vi "PMT imaging_ v1.vi"() -> ()   [LabVIEW 2012]
uses:
  <vilib>/DAQmx/write.llb/DAQmx Write (Analog 1D Wfm NChan NSamp).vi
  <vilib>/DAQmx/read.llb/DAQmx Read (Counter 1D U32 1Chan NSamp).vi
  <vilib>/DAQmx/create/channels.llb/DAQmx Create Channel (AO-Voltage-Basic).vi
  <vilib>/DAQmx/configure/timing.llb/DAQmx Timing (Sample Clock).vi
  <vilib>/DAQmx/configure/trigger.llb/DAQmx Start Trigger (Digital Edge).vi
  <vilib>/DAQmx/create/channels.llb/DAQmx Create Channel (CI-Count Edges).vi
  <vilib>/DAQmx/miscellaneous.llb/DAQmx Fill In Error Info.vi
  <resource>/objmgr/daqmx.rc
panel:
  in  "shift":i8
  in  "Normalization":dbl=255.0
  out "Output":dbl[](array[numeric])
  out "size(s)":i32
  out "data":u32[](array[numeric])
  out "Image":T1(plugin-control)
  out "Waveform Chart":dbl[](graph)
  in  "Exp Time (s)":dbl=4.0
  in  "Y line":i32=512
  in  "Y step (um)":dbl=0.1
  in  "X step (um)":dbl=0.1
  in  "X pixel":i32=512
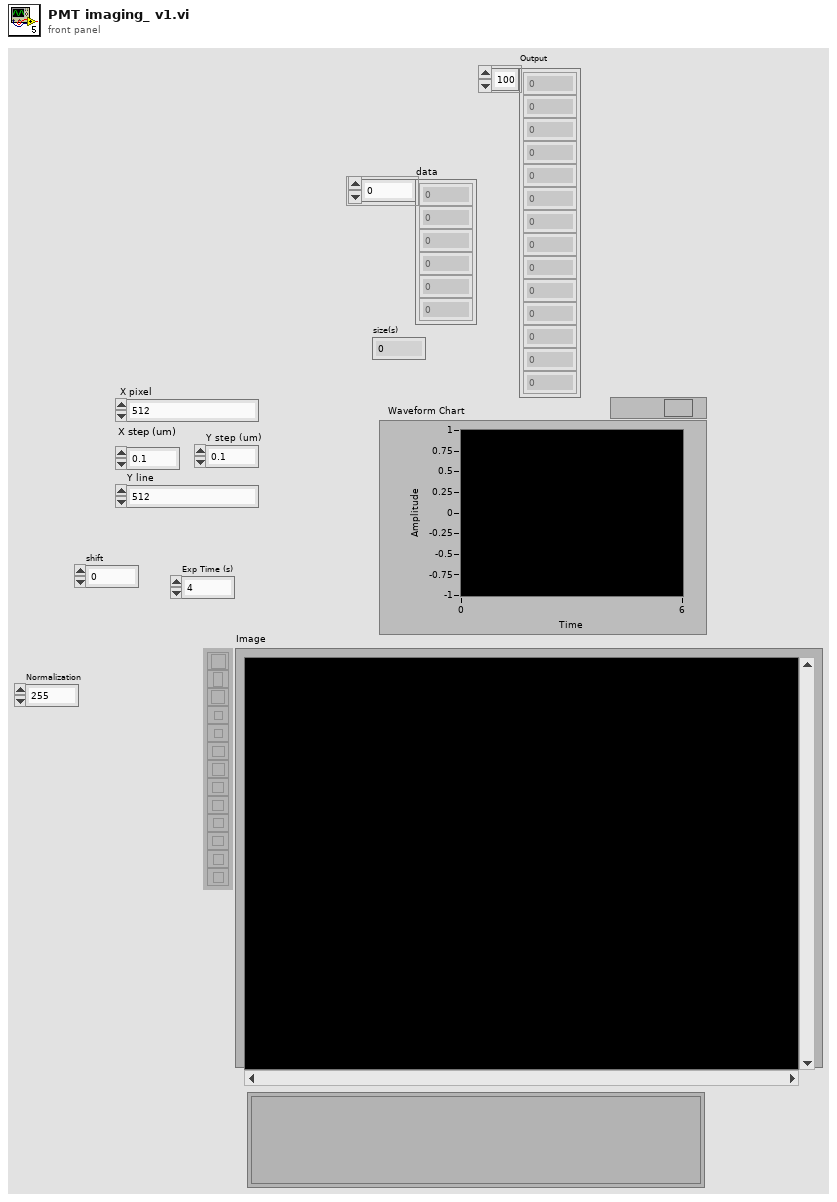
[diagram p1: front panel]
types:
  T1 = typedef "IMAQ Image.ctl" = refnum<image>
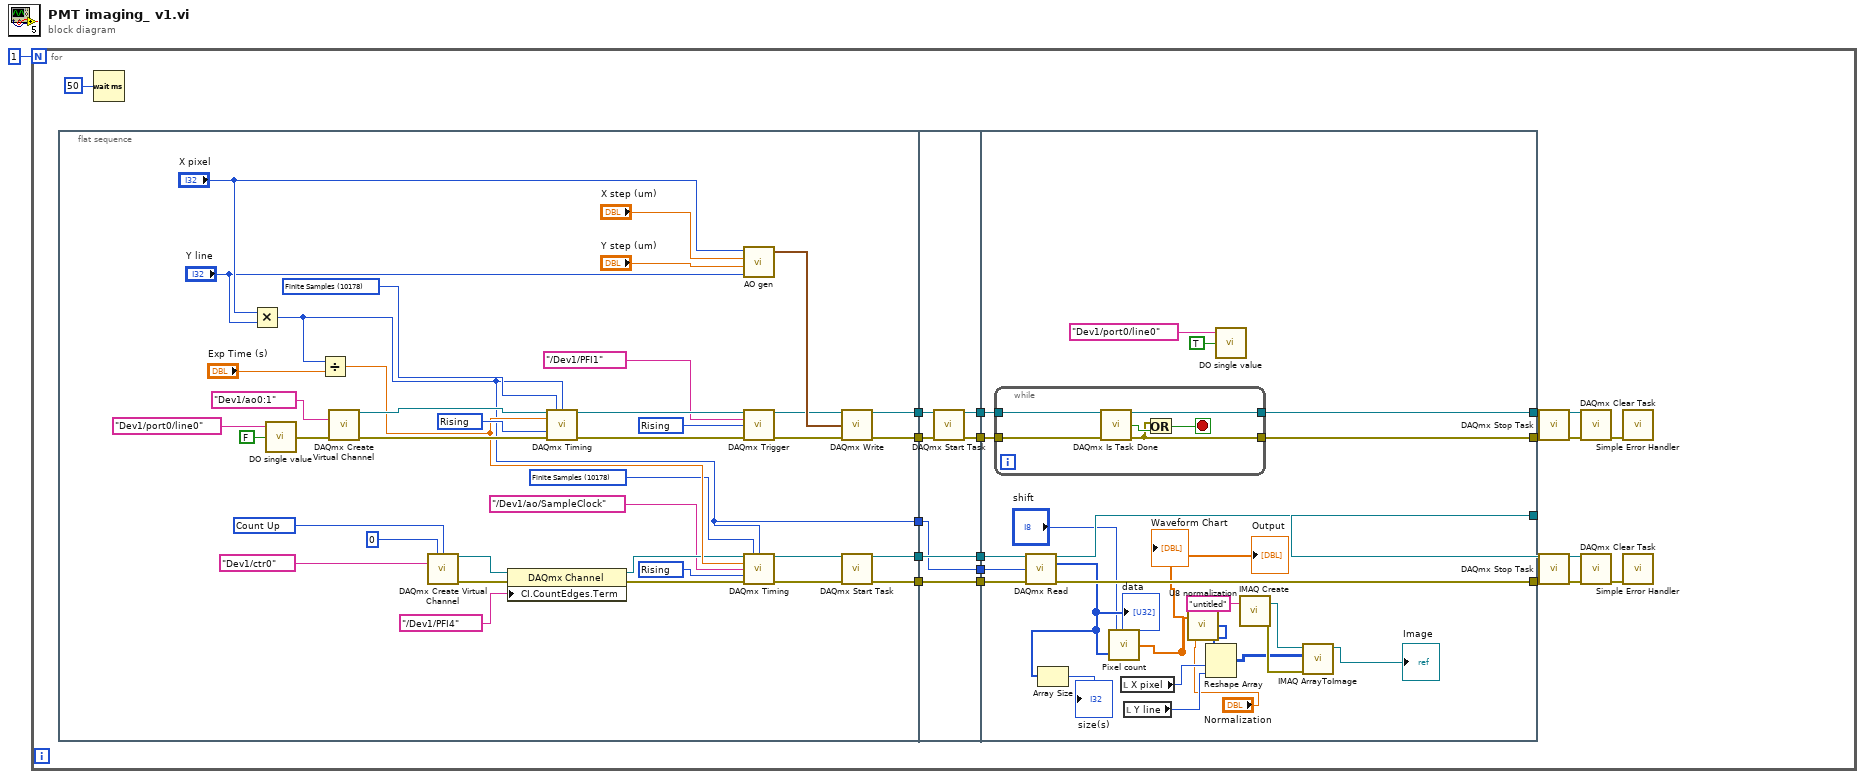
[diagram p0: block diagram]
diagram:
  n1 = for {
    N: 1 -> [_]
    n2 = flat-sequence {
      tunnel: [w44] -> w13
      tunnel: [w43] -> w12
      tunnel: [w34] -> w11
      tunnel: [w33] -> w10
      tunnel: [w32] -> w9
      tunnel: [w68] -> w6
      tunnel: [w67] -> w5
      tunnel: [w66] -> w4
      tunnel: [w65] -> w3
      tunnel: [w64] -> w2
      tunnel: w9 -> [w64]
      tunnel: w10 -> [w62]
      tunnel: w11 -> [w63]
      tunnel: w12 -> [w67]
      tunnel: w13 -> [w68]
      tunnel: [w84] -> w22
      tunnel: w6 -> [w86]
      tunnel: [w83] -> w21
      tunnel: w5 -> [w85]
      tunnel: [w90] -> w20
      tunnel: [w89] -> w19
      tunnel: w4 -> [w88]
      tunnel: w3 -> [w87]
      tunnel: w2 -> [w82]
      frame #0 {
        w24 = 10128 items=["Count Up"=10128, "Count Down"=10124, "Externally Controlled"=10326] ("count direction")
        w25 = 10280 items=["Rising"=10280, "Falling"=10171] ("edge")
        w48 = 10178 items=["Finite Samples"=10178, "Continuous Samples"=10123, "Hardware Timed Single Point"=12522] ("sample mode")
        w50 = 10280 items=["Rising"=10280, "Falling"=10171] ("active edge")
        w52 = 10178 items=["Finite Samples"=10178, "Continuous Samples"=10123, "Hardware Timed Single Point"=12522] ("sample mode")
        w56 = 10280 items=["Rising"=10280, "Falling"=10171] ("active edge")
        n3 = Multiply(x="X pixel", y="Y line") -> (x*y=w32:i32)
        n4 = call "DO single value.vi"("data"=FALSE, "lines"=tag "Dev1/port0/line0") -> ("error out"=w47:errorcluster)  [unwired: 1 in]
        n5 = Divide(x=w32, y="Exp Time (s)") -> (x/y=w49:dbl)
        n6 = call-poly <vilib>:"DAQmx Create Virtual Channel.vi"("physical channels"=tag "Dev1/ao0:1", "error in"=w47) -> ("task out"=w57:refnum<k21>, "error out"=w58:errorcluster)  [unwired: 7 in, 5 out]
        n7 = call-poly <vilib>:"DAQmx Create Virtual Channel.vi"("initial count"=u32 0, "count direction"=w24, "counter"=tag "Dev1/ctr0") -> ("task out"=w41:refnum<k21>, "error out"=w40:errorcluster)  [unwired: 4 in, 7 out]
        n8 = property class="DAQmx Channel"(reference=w41, error in=w40, "CI.CountEdges.Term"=tag "/Dev1/PFI4") -> (reference out=w38:refnum<k21>, error out=w37:errorcluster)
        n9 = call-poly <vilib>:"DAQmx Timing.vi"("task/channels in"=w57, "sample mode"=w52, "samples per channel"=w32, "rate"=w49, "active edge"=w56, "error in"=w58) -> ("task out"=w30:refnum<k21>, "error out"=w29:errorcluster)  [unwired: 1 in, 7 out]
        n10 = call "AO gen.vi"("X pixel"="X pixel", "X step (um)"="X step (um)", "Y step (um)"="Y step (um)", "Y line"="Y line") -> ("waveform output"=w51:waveform(dbl)[])  [unwired: 2 in, 1 out]
        n11 = call-poly <vilib>:"DAQmx Trigger.vi"("task/channels in"=w30, "source"=tag "/Dev1/PFI1", "edge"=w25, "error in"=w29) -> ("task out"=w28:refnum<k21>, "error out"=w27:errorcluster)  [unwired: 10 in]
        n12 = call-poly <vilib>:"DAQmx Timing.vi"("task/channels in"=w38, "sample mode"=w48, "samples per channel"=w32, "rate"=w49, "source"=tag "/Dev1/ao/SampleClock", "active edge"=w50, "error in"=w37) -> ("task out"=w36:refnum<k21>, "error out"=w35:errorcluster)  [unwired: 7 out]
        n13 = call-poly <vilib>:"DAQmx Write.vi"("task/channels in"=w28, "data"=w51, "error in"=w27) -> ("task out"=w34:refnum<k21>, "error out"=w33:errorcluster)  [unwired: 2 in, 9 out]
        n14 = call <vilib>:"DAQmx Start Task.vi"("task/channels in"=w36, "error in"=w35) -> ("task out"=w44:refnum<k21>, "error out"=w43:errorcluster)  [unwired: 12 out]
      }
      frame #1 {
        n15 = call <vilib>:"DAQmx Start Task.vi"("task/channels in"=w63, "error in"=w62) -> ("task out"=w66:refnum<k21>, "error out"=w65:errorcluster)  [unwired: 12 out]
      }
      frame #2 {
        n16 = while {
          tunnel: [w96] -> w90
          tunnel: [w95] -> w89
          tunnel: w88 -> [w94]
          tunnel: w87 -> [w93]
          stop <- w97 stop-if-true
          n17 = call <vilib>:"DAQmx Is Task Done.vi"("task/channels in"=w94, "error in"=w93) -> ("task out"=w96:refnum<k21>, "task done?"=w98:bool, "error out"=w95:errorcluster)  [unwired: 11 in]
          n18 = Or(x=w95, y=w98) -> (x .or. y?=w97:bool)
        }
        n19 = call-poly <vilib>:"DAQmx Read.vi"("task/channels in"=w86, "number of samples per channel"=w82, "error in"=w85) -> ("task out"=w84:refnum<k21>, "data"=w75:u32[], "error out"=w83:errorcluster)  [unwired: 10 in]
        "data" <- w75
        n20 = Array Size(array=w75) -> (size(s)=→"size(s)":i32)
        n21 = call "Pixel count.vi"("Input"=w75, "shift"="shift") -> ("Output"=w72:dbl[])
        "Waveform Chart" <- w72
        "Output" <- w72
        n22 = local read "X pixel"() -> (w81:i32)
        n23 = local read "Y line"() -> (w80:i32)
        n24 = call "U8 normalization.vi"("Max"="Normalization", "Input"=w72) -> ("Output"=w71:u8[])
        n25 = Reshape Array(w71, w81, w80) -> (w73:u8[][])
        n26 = call "DO single value.vi"("data"=TRUE, "lines"=tag "Dev1/port0/line0") -> ()  [unwired: 1 in, 1 out]
        n27 = call "IMAQ Create"("Image Name"="untitled") -> ("New Image"=w79:T1, "error out"=w78:errorcluster)  [unwired: 4 in]
        n28 = call "IMAQ ArrayToImage"("error in (no error)"=w78, "Image Pixels (U8)"=w73, "Image"=w79) -> ("Image Out"=→"Image":T1)  [unwired: 7 in, 1 out]
      }
    }
    n29 = Wait (ms)(milliseconds to wait=u32 50) -> ()  [unwired: 1 out]
    n30 = call <vilib>:"DAQmx Stop Task.vi"("task/channels in"=w20, "error in"=w19) -> ("task out"=w16:refnum<k21>, "error out"=w15:errorcluster)  [unwired: 12 out]
    n31 = call <vilib>:"DAQmx Stop Task.vi"("task/channels in"=w22, "error in"=w21) -> ("task out"=w17:refnum<k21>, "error out"=w18:errorcluster)  [unwired: 12 out]
    n32 = call <vilib>:"DAQmx Clear Task.vi"("task in"=w16, "error in"=w15) -> ("error out"=w8:errorcluster)  [unwired: 13 in]
    n33 = call <vilib>:"DAQmx Clear Task.vi"("task in"=w17, "error in"=w18) -> ("error out"=w7:errorcluster)  [unwired: 13 in]
    n34 = call <vilib>:"Simple Error Handler.vi"("error in (no error)"=w8) -> ()  [unwired: 4 in, 5 out]
    n35 = call <vilib>:"Simple Error Handler.vi"("error in (no error)"=w7) -> ()  [unwired: 4 in, 5 out]
  }
